vi "task9.vi"() -> ()   [LabVIEW 2017]
panel:
  out "Array":string[](array[string])
  in  "String":string
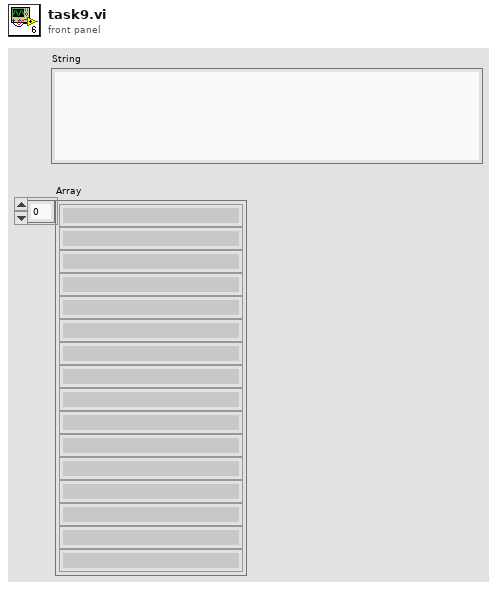
[diagram p1: front panel]
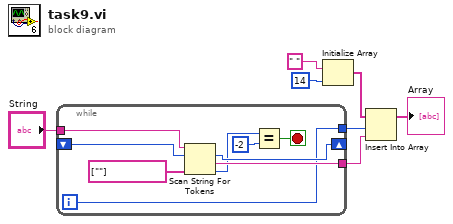
[diagram p0: block diagram]
diagram:
  n1 = while {
    tunnel: [w8] -> w4
    tunnel: [w15] -> w2
    shift-right: [w14] -> _
    shift-left: _ -> [w13]
    tunnel: "String" -> [w12]
    i -> [w8]
    stop <- w11 stop-if-true
    n2 = Scan String For Tokens(6:string[] [""] ("delimiters (\\s,\\t,\\r,\\n)"), 8:w13, 9:w12) -> (0:w10:i32, 1:w15:string, 2:w14:i32)  [unwired: 3 in, 1 out]
    n3 = Equal?(x=w10, y=-2) -> (x = y?=w11:bool)
  }
  n4 = Initialize Array(" " ("element"), 14 ("dimension size")) -> (w5:string[])
  n5 = Insert Into Array(array=w5, index=w4, new element=w2) -> (→"Array":string[])
